vi "LV to ITX XY AutoPlot.vi"(4 "X,Y Log":i32[](array[numeric]), 6 "X,Y Labels":string[](array[string])=["x label", "y label"], 8 "error in":errorcluster, 9 "Plot Names":string[](array[string]), 10 "XY-Data []":cluster{"X  array":dbl[], "Y  Array":dbl[]}[](array[cluster]), 11 "path":path=path "C:/Users/voodoo.SEAGATE/Desktop/datatest") -> (0 "error out":errorcluster, 3 "file":path=path "C:/Users/voodoo.SEAGATE/Desktop/datatest/datatest.000019.itx")   [LabVIEW 2016, in "Data.ITX.lvclass"]
doc: "Write your XY data to ITX file. This AutoPlot VI adds commands to automatically create a graph in Igor to quickly view your data.\n\n-- path: base path to save data\n-- filename: base filename\n-- Notes: add any notes here to help you remember what experiment you did\n-- XY Array: Array of Clusters (ie, Array of XY graphs)\n-- wavenames: Give each data array a unique name such as \"time, bias, current,...\"\n-- X,Y Labels: For plotting in Igor. Can be ignored.\n-- X,Y Log: Do you wan to show X or Y on Log scale in Igor?"
uses:
  Data.ITX.lvclass
  Data/Data.lvclass
panel:
  in  "command string":string="Display 'y_#wave#' vs 'x_#wave#'\nAppendToGraph 'y_#wave#' vs 'x_#wave#'\nLabel bottom \"#labelX#\"\nLabel left \"#labelY#\"\nModifyGraph rgb('y_#wave#')=(#r#,#g#,#b#)\n\\\\s('y_#wave#') #label#\nModifyGraph mirror=1\nModifyGraph width=216\nModifyGraph height={Aspect,0.6}\nModifyGraph Log(bottom)=#bottomlog#\nModifyGraph Log(left)=#leftlog#"
  in  "Notes":string
  # "Below are relevant for creating graphs in Igor"
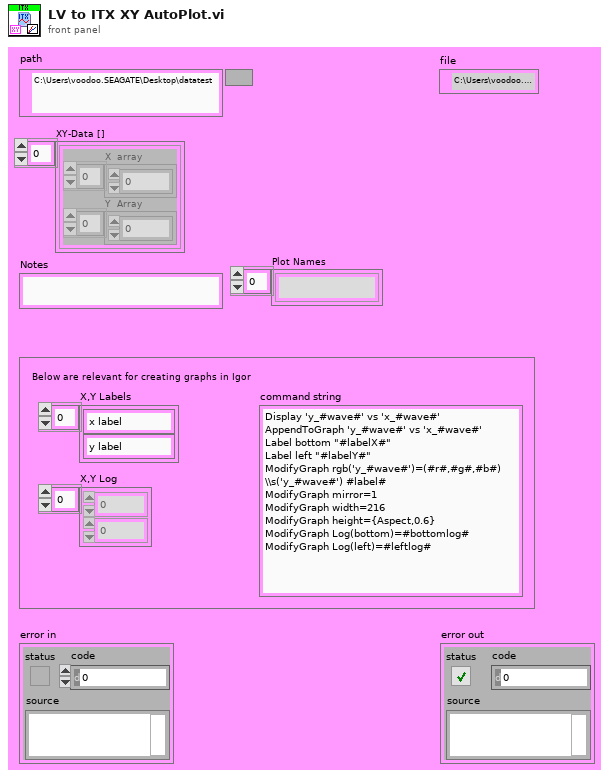
[diagram p1: front panel]
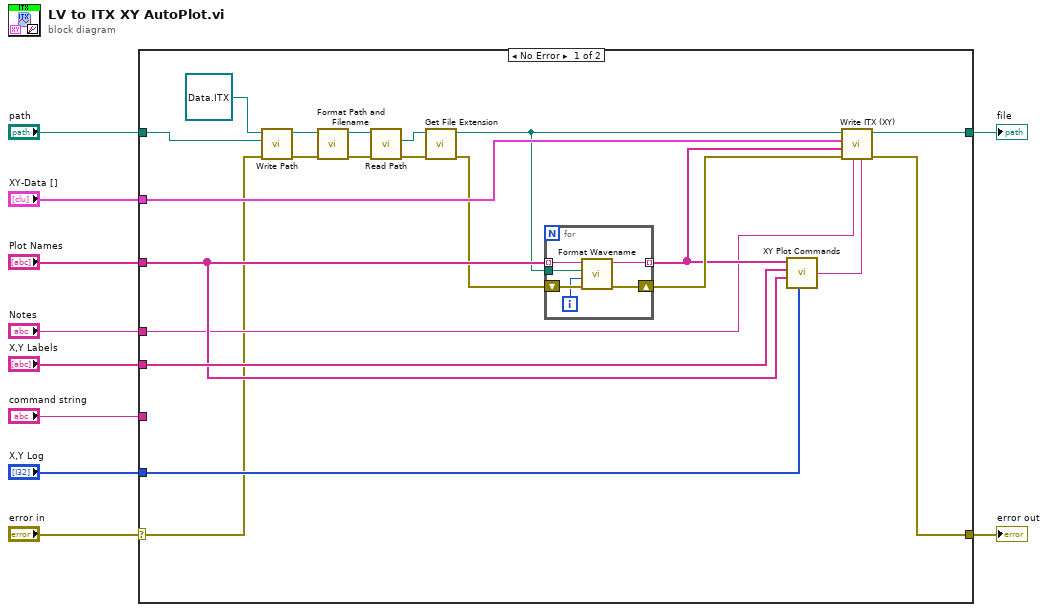
[diagram p0: block diagram]
diagram:
  n1 = case shown="No Error" "error in" {
    selector: "error in" -> [w11 w39]
    tunnel: "path" -> [w14 w38]
    tunnel: "X,Y Labels" -> [w31 _]
    tunnel: [w30 w38] -> w8
    tunnel: "X,Y Log" -> [w29 _]
    tunnel: "command string" -> [_ _]
    tunnel: "XY-Data []" -> [w28 _]
    tunnel: "Plot Names" -> [w24 _]
    tunnel: [w26 w39] -> w2
    tunnel: "Notes" -> [w22 _]
    frame No Error {
      n2 = call "Write Path.vi"("error in (no error)"=w11, "Path"=w14, "Data Save"=refnum<class "Data.ITX.lvclass"> refnum ("Data.ITX.lvclass")) -> ("error out"=w17:errorcluster, "Data Save out"=w16:refnum<class "Data.ITX.lvclass">)  [unwired: 7 in]
      n3 = call "Format Path and Filename.vi"("error in"=w17, "Data in"=w16) -> ("error out"=w18:errorcluster, "Data out"=w19:refnum<class "Data.ITX.lvclass">)  [unwired: 8 in]
      n4 = call "Read Path.vi"("error in (no error)"=w18, "Data Save"=w19) -> ("error out"=w20:errorcluster, "Path"=w21:path)  [unwired: 7 in, 1 out]
      n5 = call <vilib>:"Get File Extension.vi"("error in (no error)"=w20, "file"=w21) -> ("error out"=w12:errorcluster, "dup file"=w13:path)  [unwired: 5 in, 3 out]
      n6 = for {
        tunnel: w24 -> [w37] mode=indexing
        shift-right: [w35] -> w27
        shift-left: w12 -> [w36]
        tunnel: [w34] -> w25 mode=indexing
        tunnel: w13 -> [w32]
        i -> [w33]
        n7 = call "Format Wavename.vi"("error in (no error)"=w36, "Index"=w33, "Path"=w32, "Name"=w37) -> ("error out"=w35:errorcluster, "Formatted wavename"=w34:string)  [unwired: 6 in]
      }
      n8 = call "XY Plot Commands.vi"("X,Y Log"=w29, "Plot labels"=w24, "X,Y Labels"=w31, "wavenames"=w25) -> ("result string"=w23:string)  [unwired: 2 in]
      n9 = call "Write ITX (XY).vi"("Commands"=w23, "Notes"=w22, "error in"=w27, "wavenames"=w25, "XY Array"=w28, "filename"=w13) -> ("error out"=w26:errorcluster, "file"=w30:path)  [unwired: 4 in]
    }
    frame Error {
    }
  }
  "file" <- w8
  "error out" <- w2
